vi "string_msgbuilder.vi"(0 "?":cluster{"op":string, "topic":string}, 1 "data":string) -> ()   [LabVIEW 2014]
panel:
  out "?":T1
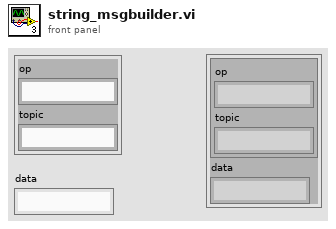
[diagram p1: front panel]
types:
  T1 = cluster{cluster{"op":string, "topic":string}, "data":string}
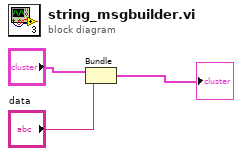
[diagram p0: block diagram]
diagram:
  n1 = Bundle("?", "data"="data") -> (→"?":T1)  [unwired: 1 in]
